vi "LED_Globals.vi"() -> ()   [LabVIEW 2019]
panel:
  in  "LED State":T1(ring)
  in  "Canifier ID":dbl=50.0
  in  "Canifier Name":string="LED_CANifier"
  # "LED States:\nTurret Locked - Solid Green\nIntaking - Solid Red\nSignal Human Player - Solid White (All 3 LED channels on)\nFiring - Flashing Green\nClimbing - Rainbow"
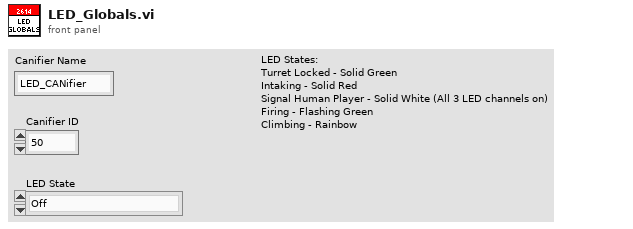
[diagram p1: front panel]
types:
  T1 = enum16{"Off", "NoOp1", "Turret Locked", "NoOp3", "Intaking", "NoOp5", "NoOp6", "Signal Human Player", "NoOp8", "NoOp9", "Firing", "NoOp11", "NoOp12", "NoOp13", "NoOp14", "Climbing - Rainbow"}
diagram:
